vi "Passing Paramters Simple Struct.vi"(8 "error in (no error)":errorcluster, 9 "radius":sgl, 10 "y":sgl, 11 "x":sgl) -> (0 "error out":errorcluster, 3 "function return":sgl)   [LabVIEW 2009, in "LabVIEWWrapper_PassingDataSampleDLL.lvlib"]
doc: "float PassingParamters_SimpleStruct (struct simpleStructCircle circle);"
uses:
  LabVIEWWrapper_PassingDataSampleDLL.lvlib
  PassingDataSampleDLL.dll
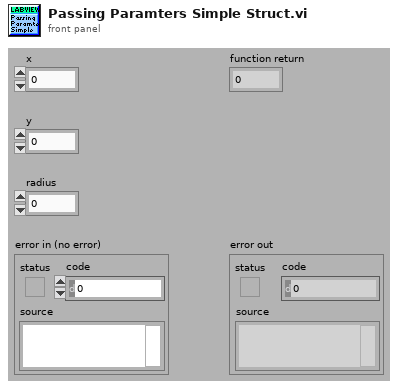
[diagram p1: front panel]
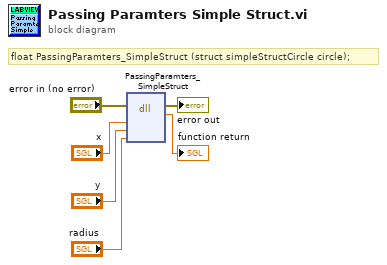
[diagram p0: block diagram]
diagram:
  # "float PassingParamters_SimpleStruct (struct simpleStructCircle circle);"
  n1 = dll-call lib="C:/My Dropbox/Systems Engineering Application/SDK/C Integration/LabVIEWWrapper/PassingDataSampleDLL.*" fn="PassingParamters_SimpleStruct"(error in="error in (no error)", "x"="x", "y"="y", "radius"="radius") -> (error out=→"error out":errorcluster, →"function return":sgl)  [unwired: 5 in, 1 out]
